vi "Core Read U8 FIFO.vi"(8 "error in (no error)":errorcluster, 9 "Timeout (ms)":i32, 11 "CIFFIFO in":refnum<class "CIF_NIChn_Fifo_U8.lvclass">) -> (0 "error out":errorcluster, 1 "timed out?":bool, 3 "CIFFIFO out":refnum<class "CIF_NIChn_Fifo_U8.lvclass">)   [LabVIEW 2021, in "CIF_NIChn_Fifo_U8.lvclass"]
uses:
  CIF_NIChn_Fifo_U8.lvclass
  CIF_NIChn_Fifo_U8.lvclass/CIF_NIChn_Fifo_U8.ctl
  CIFChannels/Typedef/Direction.ctl
  CIFChannels/CIFChannels.lvclass
  CIFChannels/Typedef/Channel State.ctl
  NIChn/CIF_NIChn.lvclass
  <vilib>/CIF Foundation/NI Channels/NIChannels.lvlib
  e6dc5e5d-6043-485e-a6bf-7c23d051166d.vi
  66a3f3ff-bc1e-4ae7-83d8-3035fbf2cfec.vi
  ChannelCommon/ChannelCommon.lvlib
  D:/dev/Packages/Channel_Manager/src/CIF_NIChn/NIChn/CIF_NIChn.lvclass
  D:/dev/Packages/Channel_Manager/src/CIFChannels/CIFChannels.lvclass
  D:/dev/Packages/Channel_Manager/src/CIF_NIChn/FIFO_U8/CIF_NIChn_Fifo_U8.lvclass
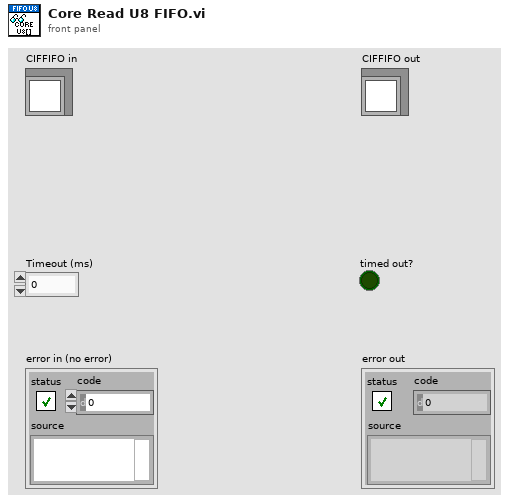
[diagram p1: front panel]
types:
  T1 = typedef "CIFChannels.lvclass/Channel State.ctl" = enum16{"Creating", "Disconnected", "Connecting", "Connected", "Destroyed"}
  T2 = typedef "CIFChannels.lvclass/Direction.ctl" = enum16{"Publisher", "Subscriber"}
  T3 = typedef "ChannelCommon.lvlib/FIFO Header.ctl" = cluster{"Length":u64, "T0":i64, "T_Out":i64, "T_Tx":i64, "Ctr":u64, "ClockID":u8}
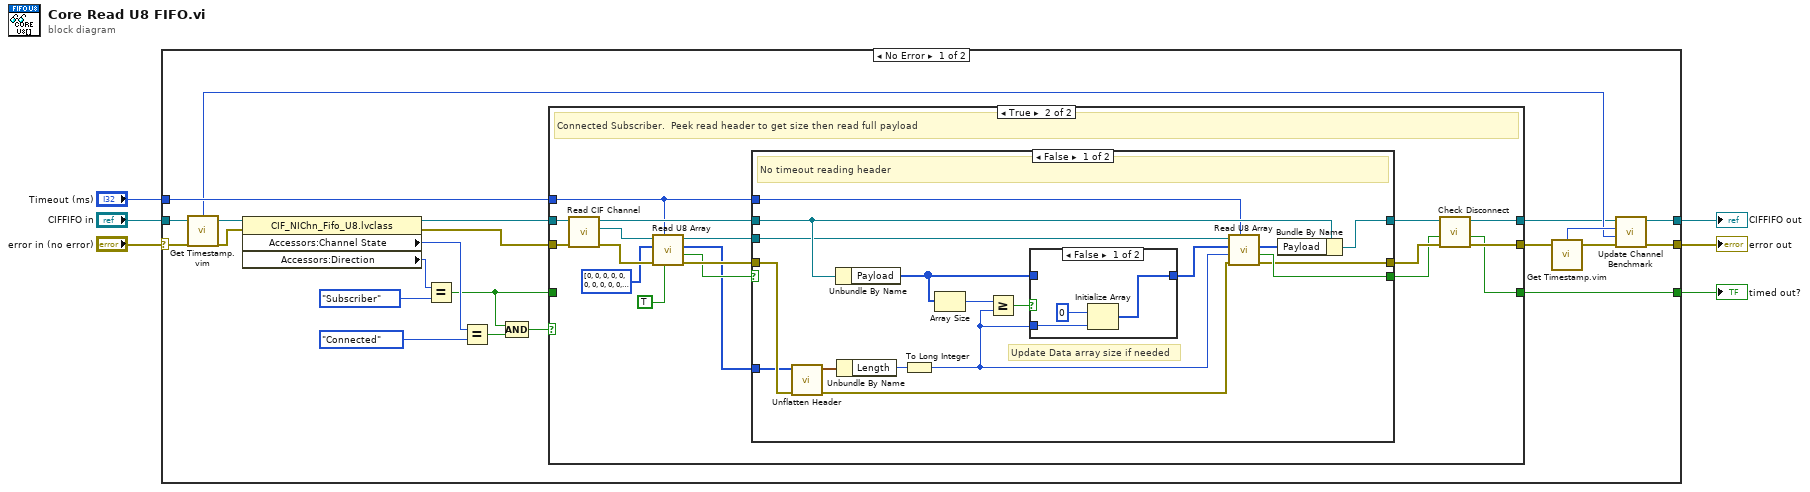
[diagram p0: block diagram]
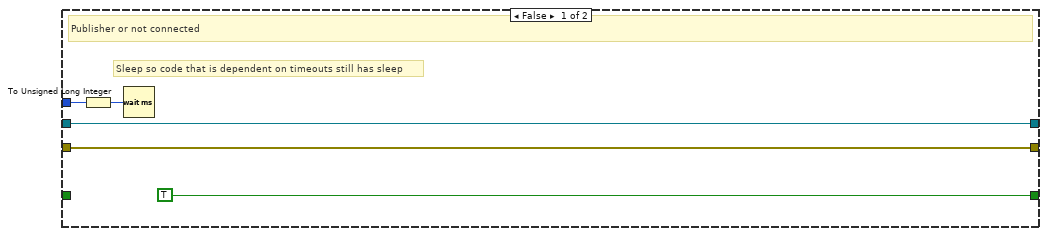
[diagram p2: hidden frame]
diagram:
  n1 = case shown="No Error" "error in (no error)" {
    selector: "error in (no error)" -> [w14 w76]
    tunnel: [w15 w76] -> w5
    tunnel: [w16 w75] -> w3
    tunnel: "CIFFIFO in" -> [w13 w75]
    tunnel: [w27 _] -> w2
    tunnel: "Timeout (ms)" -> [w17 _]
    frame No Error {
      n2 = call "Get Timestamp.vim"("Anything in"=w13) -> ("Time (ns)"=w10:i64, "Anything out"=w12:refnum<class "CIF_NIChn_Fifo_U8.lvclass">)  [unwired: 2 in]
      n3 = property class="CIF_NIChn_Fifo_U8.lvclass"(reference=w12, error in=w14) -> (reference out=w26:refnum<class "CIF_NIChn_Fifo_U8.lvclass">, error out=w25:errorcluster, "Accessors:Channel State"=w22:T1, "Accessors:Direction"=w24:T2)
      n4 = Equal?(x=w24, y=Direction."Subscriber") -> (x = y?=w18:bool)
      n5 = Equal?(x=w22, y=Channel_State."Connected") -> (x = y?=w20:bool)
      n6 = Compound Arithmetic op=AND(w18, w20) -> (w19:bool)
      n7 = case shown="True" w19 {
        tunnel: [TRUE ("timeout out") w43] -> w27
        tunnel: w25 -> [w31 w49]
        tunnel: w26 -> [w32 w50]
        tunnel: w18 -> [_ _]
        tunnel: [w32 w48] -> w8
        tunnel: [w31 w47] -> w7
        tunnel: w17 -> [w29 w34]
        frame False {
          # "Sleep so code that is dependent on timeouts still has sleep"
          # "Publisher or not connected"
          n8 = To Unsigned Long Integer(number=w29) -> (unsigned 32bit integer=w28:u32)
          n9 = Wait (ms)(milliseconds to wait=w28) -> ()  [unwired: 1 out]
        }
        frame True {
          # "Connected Subscriber.  Peek read header to get size then read full payload"
          n10 = call "Read CIF Channel.vi"("error in (no error)"=w49, "CIFTag in"=w50) -> ("error out"=w44:errorcluster, "CIF Channel"=w45:refnum<k21>, "CIFTag out"=w46:refnum<class "CIF_NIChn_Fifo_U8.lvclass">)  [unwired: 7 in]
          n11 = call <vilib>:"Read U8 Array.vi"("Peek?"=TRUE, "Timeout (ms)"=w34, "error in"=w44, "U8 Array in"=u8[] [0, 0, 0, 0, 0, 0, 0, 0, 0, 0, 0, 0, 0, 0, 0, 0, 0, 0, 0, 0, 0, 0, 0, 0, 0, 0, 0, 0, 0, 0, 0, 0, 0, 0, 0, 0, 0, 0, 0, 0, 0, 0, 0, 0, 0, 0, 0, 0], "CIF Channel in"=w45) -> ("error out"=w41:errorcluster, "Timed out?"=w36:bool, "U8 Array out"=w33:u8[], "CIF Channel out"=w42:refnum<k21>)  [unwired: 3 in]
          n12 = case shown="False" w36 {
            selector: w36 -> [_ w74]
            tunnel: w46 -> [w67 w73]
            tunnel: w42 -> [w66 _]
            tunnel: w41 -> [w62 w72]
            tunnel: w33 -> [w60 _]
            tunnel: [w51 w72] -> w38
            tunnel: [w53 w73] -> w37
            tunnel: [w52 w74] -> w35
            tunnel: w34 -> [w63 _]
            frame False {
              # "Update Data array size if needed"
              # "No timeout reading header"
              n13 = call "Unflatten Header.vi"("error in (no error)"=w62, "Flattened Data in"=w60) -> ("error out"=w61:errorcluster, "Header out"=w65:T3)  [unwired: 7 in, 1 out]
              n14 = Unbundle By Name(w67) -> ("Payload"=w55:u8[])
              n15 = Unbundle By Name(w65) -> ("Length"=w64:u64)
              n16 = To Long Integer(number=w64) -> (32bit integer=w56:i32)
              n17 = Array Size(array=w55) -> (size(s)=w57:i32)
              n18 = Greater Or Equal?(x=w57, y=w56) -> (x >= y?=w58:bool)
              n19 = case shown="False" w58 {
                tunnel: w55 -> [_ w71]
                tunnel: [w70 w71] -> w54
                tunnel: w56 -> [w68 _]
                frame False {
                  n20 = Initialize Array(u8 0, w68) -> (w70:u8[])
                }
                frame True {
                }
              }
              n21 = call <vilib>:"Read U8 Array.vi"("Timeout (ms)"=w63, "error in"=w61, "Number of Elements"=w56, "U8 Array in"=w54, "CIF Channel in"=w66) -> ("error out"=w51:errorcluster, "Timed out?"=w52:bool, "U8 Array out"=w59:u8[])  [unwired: 3 in, 1 out]
              n22 = Bundle By Name(cluster=w67, "Payload"=w59) -> (w53:refnum<class "CIF_NIChn_Fifo_U8.lvclass">)
            }
            frame True {
              # "Timeout reading header"
            }
          }
          n23 = call "Check Disconnect.vi"("error in (no error)"=w38, "timeout in"=w35, "CIFTag in"=w37) -> ("error out"=w47:errorcluster, "timeout out"=w43:bool, "CIFTag out"=w48:refnum<class "CIF_NIChn_Fifo_U8.lvclass">)  [unwired: 5 in, 1 out]
        }
      }
      n24 = call "Get Timestamp.vim"("Anything in"=w7) -> ("Time (ns)"=w11:i64, "Anything out"=w9:errorcluster)  [unwired: 2 in]
      n25 = call "Update Channel Benchmark.vi"("error in (no error)"=w9, "X0"=w10, "X1"=w11, "CIFChannels in"=w8) -> ("error out"=w15:errorcluster, "CIFChannels out"=w16:refnum<class "CIF_NIChn_Fifo_U8.lvclass">)  [unwired: 6 in]
    }
    frame Error {
    }
  }
  "error out" <- w5
  "CIFFIFO out" <- w3
  "timed out?" <- w2
